vi "Zero Accelerometer.vi"(8 "error in (no error)":errorcluster) -> (0 "error out":errorcluster, 2 "Accelerometer Data out":T1)   [LabVIEW 2013]
doc: "Use this template to build a VI to use as a subVI."
uses:
  Accelerometer Data.ctl
panel:
  in  "reset":bool
  in  "time":u64
  in  "Accelerometer Data in":T1
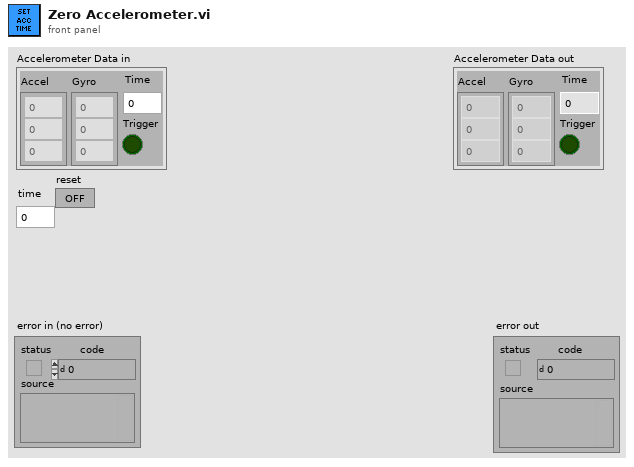
[diagram p1: front panel]
types:
  T1 = typedef "Accelerometer Data.ctl" = cluster{"Accel":dbl[], "Gyro":dbl[], "Time":u64, "Trigger":bool}
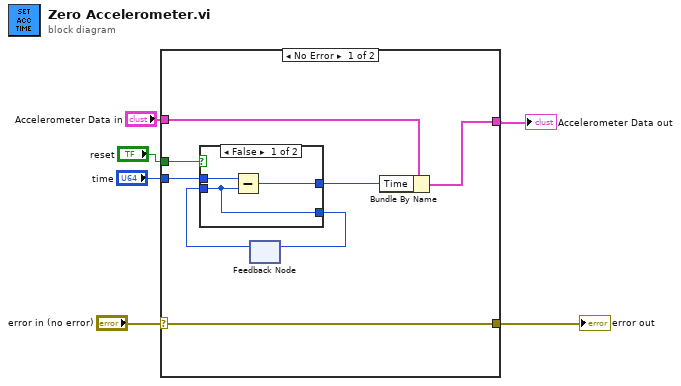
[diagram p0: block diagram]
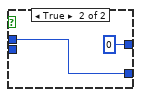
[diagram p2: hidden frame]
diagram:
  n1 = case shown="No Error" "error in (no error)" {
    selector: "error in (no error)" -> [w7 w21]
    tunnel: [w7 w21] -> w5
    tunnel: "Accelerometer Data in" -> [w14 w20]
    tunnel: "time" -> [w13 _]
    tunnel: "reset" -> [w10 _]
    tunnel: [w8 w20] -> w1
    frame No Error {
      n2 = feedback #1() -> (w11:u64)  [unwired: 1 in]
      n3 = case shown="False" w10 {
        tunnel: w13 -> [w17 w19]
        tunnel: w11 -> [w16 _]
        tunnel: [w16 w19] -> w12
        tunnel: [w15 u64 0] -> w9
        frame False {
          n4 = Subtract(x=w17, y=w16) -> (x-y=w15:u64)
        }
        frame True {
        }
      }
      n5 = feedback-in #1(w12) -> ()
      n6 = Bundle By Name(cluster=w14, "Time"=w9) -> (w8:T1)
    }
    frame Error {
    }
  }
  "error out" <- w5
  "Accelerometer Data out" <- w1
